vi "(SubVI)System Command_LDO Control.vi"(8 "error in (no error)":errorcluster caption="에러 입력(에러 없음)", 10 "T : On":bool, 11 "LDO":T1) -> (0 "error out":errorcluster caption="에러 출력", 3 "Read Data":u8[](array[numeric]))   [LabVIEW 2020]
uses:
  Controls/(Ctrl)System Command_LDO.ctl
  Serial/Controls/(Ctrl)Serial_Write Read Option.ctl
  Serial/Instance VIs/(SubVI)Serial_Write-Read.vi
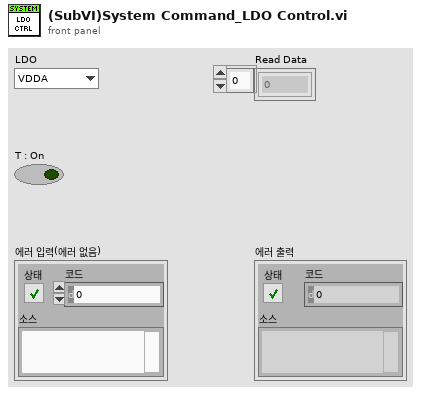
[diagram p1: front panel]
types:
  T1 = typedef "(Ctrl)System Command_LDO.ctl" = enum8{"VDDA", "VDDM", "VDDA_ADJ", "VDDM_ADJ", "VDDIO"}
  T2 = typedef "(Ctrl)Serial_Write Read Option.ctl" = cluster{"Echo Request":bool, "Header Verification":bool, "Checksum Verification":bool, "User Code Verifiaction":bool}
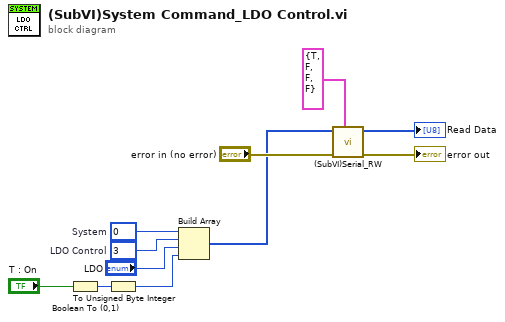
[diagram p0: block diagram]
diagram:
  w9 = u8 3  # LDO Control
  w10 = u8 0  # System
  n1 = Boolean To (0,1)(Boolean="T : On") -> (0, 1=w3:i16)
  n2 = To Unsigned Byte Integer(number=w3) -> (unsigned 8bit integer=w2:u8)
  n3 = Build Array(w10, w9, "LDO", w2) -> (w1:u8[])
  n4 = call-poly "(SubVI)Serial_RW.vi"("Option"=T2 {"Echo Request"=TRUE, "Header Verification"=FALSE, "Checksum Verification"=FALSE, "User Code Verifiaction"=FALSE}, "error in (no error)"="error in (no error)", "Data to Write"=w1) -> ("error out"=→"error out":errorcluster, "Read Data"=→"Read Data":u8[])  [unwired: 6 in, 1 out]
